vi "Pose to Transformation Matrix.vi"(8 "error in (no error)":errorcluster, 11 "Pose":T2) -> (0 "error out":errorcluster, 3 "Transformation Matrix":T1)   [LabVIEW 2020, in "g_ar_toolkit.ar.lvlib"]
uses:
  g_ar_toolkit.ar.lvlib
  Pose.ctl
  rvec.ctl
  g_ar_toolkit.common/tvec.ctl
  <vilib>/Analysis/Matrix/Datatypes/RealMatrix.ctl
  RodriguesRVecToRMat.vi
  <vilib>/Analysis/Matrix/Numeric/Conversions/Array To Matrix.vi
  <vilib>/Analysis/Matrix/Numeric/Conversions/Array To Matrix - RA2.vi
  <vilib>/Utility/error.llb/Error Cluster From Error Code.vi
  <vilib>/Analysis/Matrix/NI_Matrix.lvlib
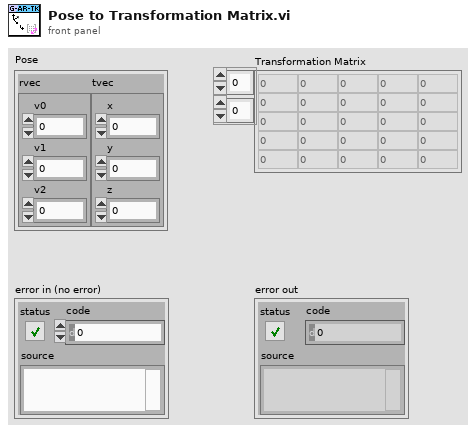
[diagram p1: front panel]
types:
  T1 = typedef "NI_Matrix.lvlib/RealMatrix.ctl" = dbl[][]
  T2 = typedef "g_ar_toolkit.ar.lvlib/Pose.ctl" = cluster{"rvec":T3, "tvec":T4}
  T3 = typedef "g_ar_toolkit.ar.lvlib/rvec.ctl" = cluster{"v0":dbl, "v1":dbl, "v2":dbl}
  T4 = typedef "g_ar_toolkit.ar.lvlib/tvec.ctl" = cluster{"x":dbl, "y":dbl, "z":dbl}
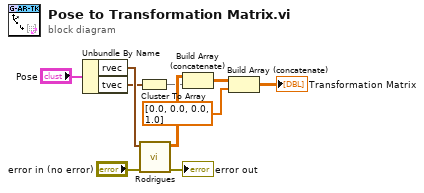
[diagram p0: block diagram]
diagram:
  n1 = Unbundle By Name("Pose") -> ("rvec"=w9:T3, "tvec"=w6:T4)
  n2 = Cluster To Array(cluster=w6) -> (array=w7:dbl[])
  n3 = call-poly "Rodrigues.vi"("error in (no error)"="error in (no error)", "rvec"=w9) -> ("error out"=→"error out":errorcluster, "Rotation Matrix"=w8:T1)  [unwired: 8 in]
  n4 = Build Array (concatenate)(w8, w7) -> (w3:T1)
  n5 = Build Array (concatenate)(w3, dbl[] [0.0, 0.0, 0.0, 1.0]) -> (→"Transformation Matrix":T1)
